vi "lab2qn1.vi"() -> ()   [LabVIEW 2025]
uses:
  <vilib>/measure/NI_MABase.lvlib
panel:
  in  "Numeric 2":dbl
  in  "Numeric":dbl
  out "Waveform Chart":waveform(dbl)(graph)
  out "Waveform Graph":waveform(dbl)(graph)
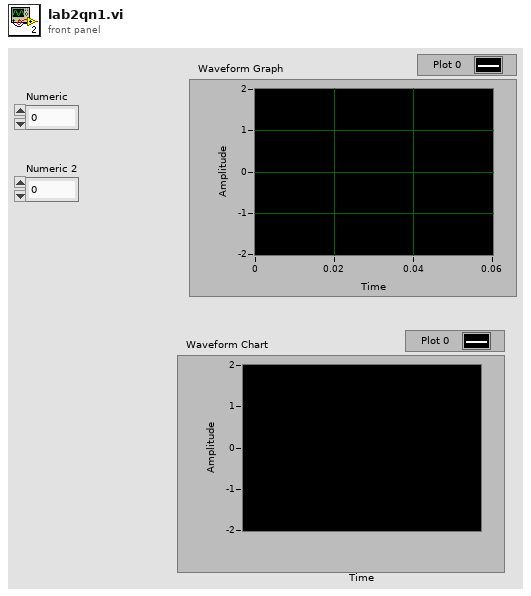
[diagram p1: front panel]
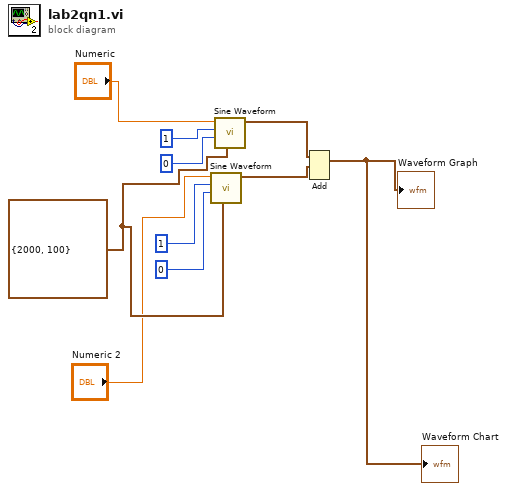
[diagram p0: block diagram]
diagram:
  w3 = cluster{i32, i32} {2000, 100}
  n1 = call <vilib>:"Sine Waveform.vi"("sampling info"=w3, "phase"=0, "amplitude"=1, "frequency"="Numeric 2") -> ("signal out"=w9:waveform(dbl))  [unwired: 6 in, 1 out]
  n2 = call <vilib>:"Sine Waveform.vi"("sampling info"=w3, "phase"=0, "amplitude"=1, "frequency"="Numeric") -> ("signal out"=w10:waveform(dbl))  [unwired: 6 in, 1 out]
  n3 = Add(1:w9, 2:w10) -> (0:→"Waveform Graph" →"Waveform Chart":waveform(dbl))  [unwired: 1 in, 1 out]
